vi "GetClassPath.vi"(8 "error in (no error)":errorcluster caption="entrée d'erreur (pas d'erreur)", 11 "ClassName":string) -> (0 "error out":errorcluster caption="sortie d'erreur", 2 "IsInstrument":bool, 3 "ClassPath":path)   [LabVIEW 2019]
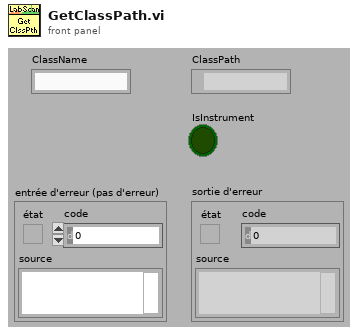
[diagram p1: front panel]
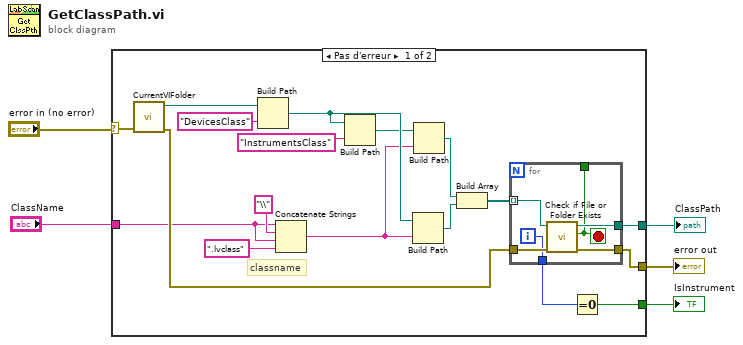
[diagram p0: block diagram]
diagram:
  n1 = case shown="Pas d'erreur" "error in (no error)" {
    selector: "error in (no error)" -> [w10 w30]
    tunnel: "ClassName" -> [w6 _]
    tunnel: [w9 _] -> w3
    tunnel: [w8 w30] -> w2
    tunnel: [w7 _] -> w1
    frame No Error {
      # "classname"
      n2 = call <userlib>:"CurrentVIFolder.vi"("error in (no error)"=w10) -> ("error out"=w23:errorcluster, "Chemin"=w22:path)  [unwired: 8 in, 1 out]
      n3 = Build Path(base path=w22, name or relative path="DevicesClass" ("chaîne")) -> (appended path=w17:path)
      n4 = Concatenate Strings(w6, "\\" ("chaîne"), w6, ".lvclass" ("chaîne")) -> (w15:string)
      n5 = Build Path(base path=w17, name or relative path="InstrumentsClass" ("nom ou chemin relatif")) -> (appended path=w16:path)
      n6 = Build Path(base path=w17, name or relative path=w15) -> (appended path=w13:path)
      n7 = Build Path(base path=w16, name or relative path=w15) -> (appended path=w14:path)
      n8 = Build Array(w14, w13) -> (w12:path[])
      n9 = for {
        tunnel: [w29] -> w9
        tunnel: [w28] -> w8
        tunnel: w23 -> [w27]
        tunnel: [w26] -> _
        tunnel: w12 -> [w25] mode=indexing
        tunnel: [w24] -> w11
        i -> [w24]
        stop <- w26 stop-if-true
        n10 = call <vilib>:"Check if File or Folder Exists.vi"("error in (no error)"=w27, "path"=w25) -> ("error out"=w28:errorcluster, "file or folder exists?"=w26:bool, "dup path"=w29:path)  [unwired: 7 in]
      }
      n11 = Equal To 0?(x=w11) -> (x = 0?=w7:bool)
    }
    frame Error {
    }
  }
  "error out" <- w2
  "IsInstrument" <- w1
  "ClassPath" <- w3
